vi "Get Subscribers.vi"(8 "error in (no error)":errorcluster, 10 "Topic":string, 11 "Broadcaster in":refnum<class "BroadcastBroker.lvclass">) -> (0 "error out":errorcluster, 2 "Subscribers":string[](array[string]), 3 "Broadcaster out":refnum<class "BroadcastBroker.lvclass">)   [LabVIEW 2015, in "BroadcastBroker.lvclass"]
uses:
  BroadcastBroker.lvclass
  BroadcastBroker.lvclass/BroadcastBroker.ctl
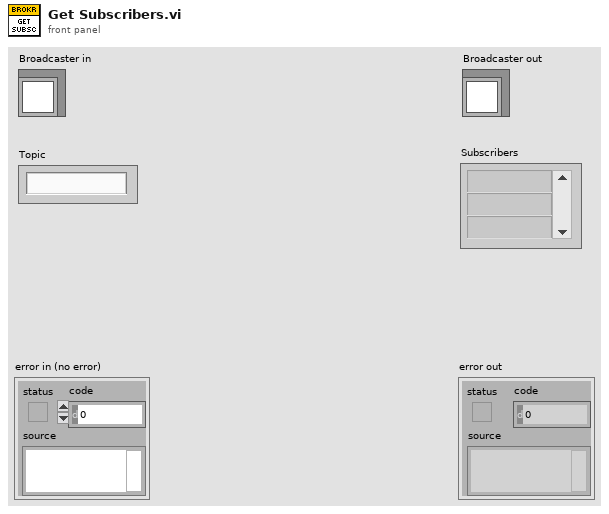
[diagram p1: front panel]
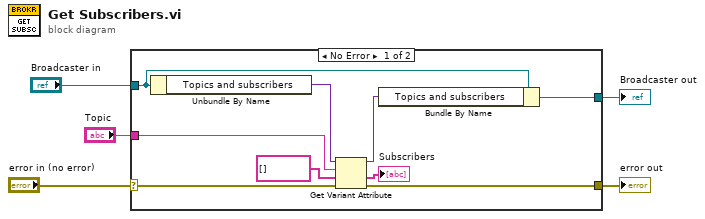
[diagram p0: block diagram]
diagram:
  n1 = case shown="No Error" "error in (no error)" {
    selector: "error in (no error)" -> [w12 w16]
    tunnel: [w9 w16] -> w4
    tunnel: [w7 w15] -> w2
    tunnel: "Broadcaster in" -> [w14 w15]
    tunnel: "Topic" -> [w10 _]
    frame No Error {
      n2 = Unbundle By Name(w14) -> ("Topics and subscribers"=w13:variant)
      n3 = Get Variant Attribute(Variant=w13, name=w10, default value (empty Variant)=string[] [], error in=w12) -> (duplicate Variant=w8:variant, value=→"Subscribers":string[], error out=w9:errorcluster)  [unwired: 1 out]
      n4 = Bundle By Name(cluster=w14, "Topics and subscribers"=w8) -> (w7:refnum<class "BroadcastBroker.lvclass">)
    }
    frame Error {
    }
  }
  "error out" <- w4
  "Broadcaster out" <- w2
